vi "semaforo.vi"() -> ()   [LabVIEW 2016]
panel:
  out "Waveform Chart 6":dbl(graph)
  in  "Stop Button 6":bool
  out "Numeric Control 6":i32
  out "Waveform Chart 5":dbl(graph)
  in  "Stop Button 5":bool
  out "Numeric Control 5":i32
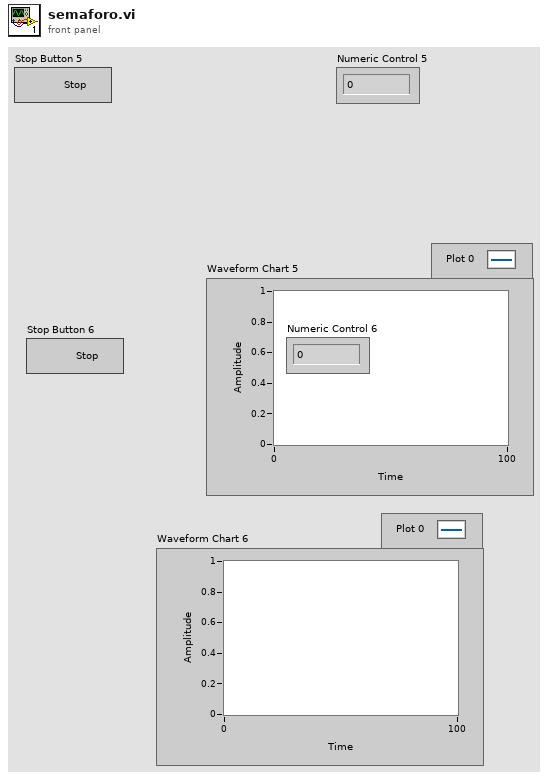
[diagram p1: front panel]
types:
  T1 = typedef "Semaphore RefNum" = refnum<k1>
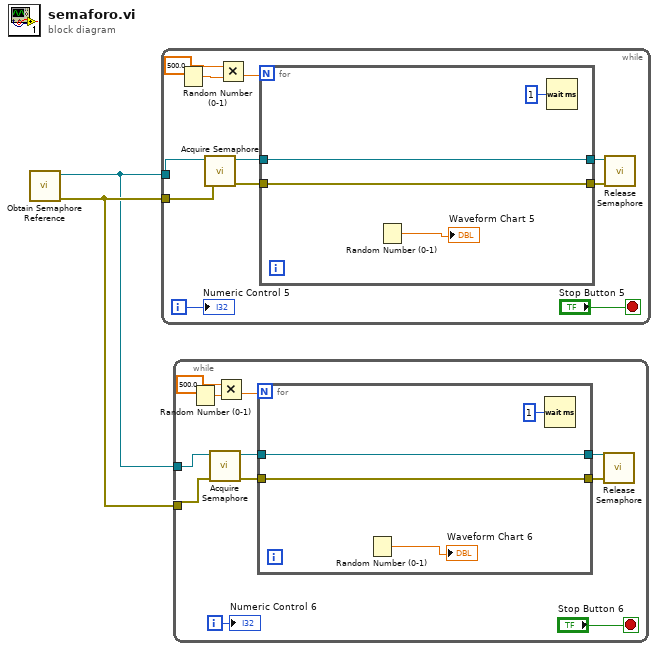
[diagram p0: block diagram]
diagram:
  n1 = call <vilib>:"Obtain Semaphore Reference.vi"() -> ("error out"=w2:errorcluster, "semaphore"=w1:T1)  [unwired: 5 in, 1 out]
  n2 = while {
    tunnel: w1 -> [w7]
    tunnel: w2 -> [w8]
    i -> [w9]
    stop <- "Stop Button 5" stop-if-true
    n3 = Random Number (0-1)() -> (number: 0 to 1=w13:dbl)
    n4 = call <vilib>:"Acquire Semaphore.vi"("error in (no error)"=w8, "semaphore"=w7) -> ("error out"=w5:errorcluster, "semaphore out"=w6:T1)  [unwired: 3 in, 1 out]
    n5 = Multiply(x=500.0, y=w13) -> (x*y=w11:dbl)
    n6 = for {
      N: w11 -> [_]
      tunnel: [w15] -> w3
      tunnel: w6 -> [w15]
      tunnel: [w14] -> w4
      tunnel: w5 -> [w14]
      n7 = Random Number (0-1)() -> (number: 0 to 1=→"Waveform Chart 5":dbl)
      n8 = Wait (ms)(milliseconds to wait=u32 1) -> ()  [unwired: 1 out]
    }
    n9 = call <vilib>:"Release Semaphore.vi"("error in (no error)"=w4, "semaphore"=w3) -> ()  [unwired: 4 in, 2 out]
    "Numeric Control 5" <- w9
  }
  n10 = while {
    tunnel: w2 -> [w23]
    tunnel: w1 -> [w22]
    i -> [w24]
    stop <- "Stop Button 6" stop-if-true
    n11 = Random Number (0-1)() -> (number: 0 to 1=w28:dbl)
    n12 = call <vilib>:"Acquire Semaphore.vi"("error in (no error)"=w23, "semaphore"=w22) -> ("error out"=w20:errorcluster, "semaphore out"=w21:T1)  [unwired: 3 in, 1 out]
    n13 = Multiply(x=500.0, y=w28) -> (x*y=w26:dbl)
    n14 = for {
      N: w26 -> [_]
      tunnel: [w30] -> w18
      tunnel: w21 -> [w30]
      tunnel: [w29] -> w19
      tunnel: w20 -> [w29]
      n15 = Random Number (0-1)() -> (number: 0 to 1=→"Waveform Chart 6":dbl)
      n16 = Wait (ms)(milliseconds to wait=u32 1) -> ()  [unwired: 1 out]
    }
    n17 = call <vilib>:"Release Semaphore.vi"("error in (no error)"=w19, "semaphore"=w18) -> ()  [unwired: 4 in, 2 out]
    "Numeric Control 6" <- w24
  }
